vi "SlideBoundsRead.vi"(4 "error in (no error)":errorcluster, 6 "Container State":T2, 7 "Display State In":T1) -> (0 "error out":errorcluster, 2 "Value":cluster{"min":i16, "max":i16}, 3 "Display State Out":T1)   [LabVIEW 2019, in "XVerticalSlide.xctl"]
uses:
  XVerticalSlide.xctl
  <vilib>/_xctls/Container State.ctl
  State.ctl
  <vilib>/_xctls/XControlSupport.lvlib
panel:
  # "Replace the Value Indicator below with an Indicator of desired type.\nDo not remove this Indicator or the others from the connector pane. \nDo not change the connector pane pattern.\nThe Value Indicator should always be the second terminal from top on the output side in the connector pane."
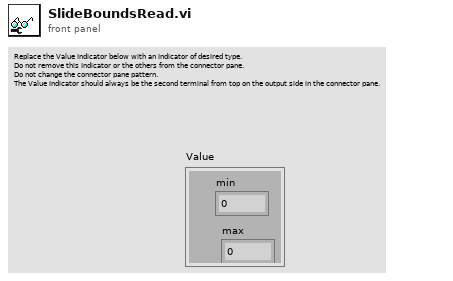
[diagram p1: front panel]
types:
  T1 = typedef "XVerticalSlide.xctl/State.ctl" = cluster{"low":i16, "high":i16, "min":i16, "max":i16}
  T2 = typedef "XControlSupport.lvlib/Container State.ctl" = cluster{"Indicator?":bool, "Run Mode?":bool, " Refnum":refnum<vi>}
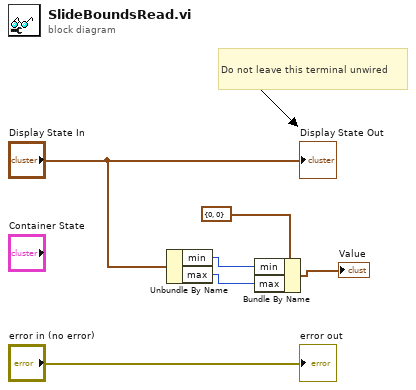
[diagram p0: block diagram]
diagram:
  # "Do not leave this terminal unwired"
  n1 = Unbundle By Name("Display State In") -> ("min"=w5:i16, "max"=w2:i16)
  n2 = Bundle By Name(cluster=cluster{"min":i16, "max":i16} {"min"=0, "max"=0} ("Value 2"), "min"=w5, "max"=w2) -> (→"Value":cluster{"min":i16, "max":i16})
  "error out" <- "error in (no error)"
  "Display State Out" <- "Display State In"
